vi "Analog Read Benchmark.vi"(0 "Stop Button":bool, 11 "AO Channels":u8[](array[numeric])=[0, 0, 0, 0, 0, 0, 0, 0, 0, 0, 0, 0]) -> (2 "Voltages":dbl[](array[numeric]), 3 "Loop Time (ms)":i32, 6 "Loop Rate":dbl(graph), 7 "Device Name":string)   [LabVIEW 2013]
uses:
  <vilib>/LabVIEW Hacker/LINX/Private/Type Defs/Interface.ctl
  <vilib>/LabVIEW Hacker/LINX/Private/Device/Type Defs/TCP Config.ctl
  <vilib>/LabVIEW Hacker/LINX/Private/Device/Device.lvlib
  <vilib>/LabVIEW Hacker/LINX/LVH-LINX.lvlib
  <vilib>/ptbypt/NI_PtbyPt.lvlib
panel:
  out "Voltages":dbl[](graph)
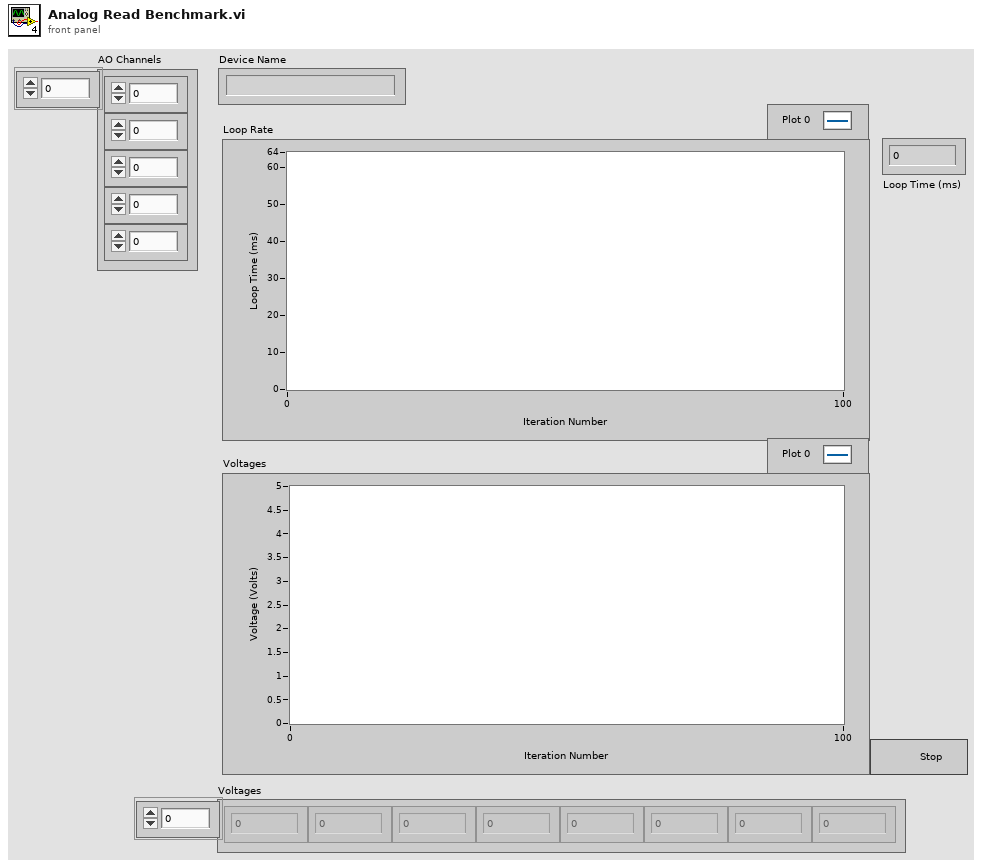
[diagram p1: front panel]
types:
  T1 = typedef "LVH-LINX.lvlib/Device.lvlib/TCP Config.ctl" = cluster{"IP Address":string, "Port":u16}
  T2 = typedef "LVH-LINX.lvlib/Interface.ctl" = enum16{"Serial", "TCP"}
  T3 = typedef "LVH-LINX.lvlib/Device.lvlib/LINX Device Config.ctl" = cluster{"Interface":T2, "COM Port":refnum<visa-resource-name>, "TCP Configuration":T1, "Device Family":T4, "Device ID":u8, "Device Name":string, "TCP Ref":refnum<k5>}
  T4 = typedef "LVH-LINX.lvlib/Device Family.ctl" = enum8{"National Instruments", "Digilent", "Arduino"}
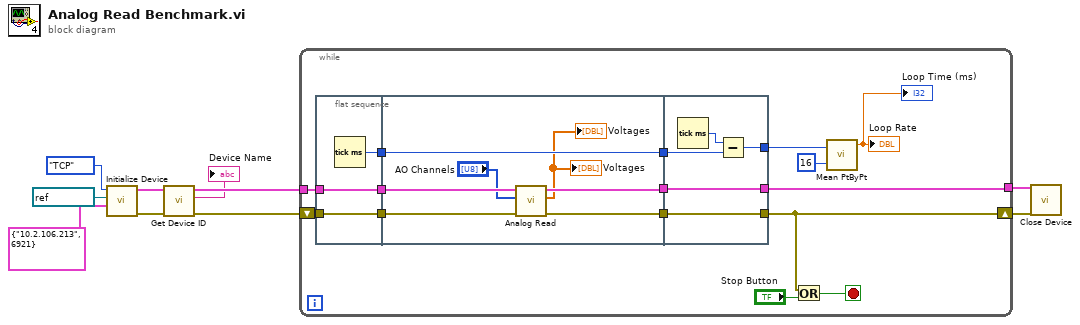
[diagram p0: block diagram]
diagram:
  n1 = call <vilib>:"Initialize Device.vi"("TCP Configuration"=T1 {"IP Address"="10.2.106.213", "Port"=6921}, "COM Port"=refnum<visa-resource-name> "COM5", "Interface"=Interface."TCP") -> ("Error Out"=w6:errorcluster, "LINX Device Config"=w7:T3)  [unwired: 6 in, 1 out]
  n2 = call <vilib>:"Get Device ID.vi"("Error In"=w6, "LINX Device Config"=w7) -> ("Error Out"=w5:errorcluster, "Device Name"=→"Device Name":string, "LINX Device Config"=w4:T3)  [unwired: 7 in]
  n3 = while {
    tunnel: w4 -> [w25]
    shift-right: [w11] -> w8
    shift-left: w5 -> [w13]
    tunnel: [w16] -> w2
    stop <- w24 stop-if-true
    n4 = flat-sequence {
      tunnel: w25 -> [w28]
      tunnel: [w28] -> w22
      tunnel: [w27] -> w21
      tunnel: w13 -> [w26]
      tunnel: [w26] -> w12
      tunnel: w22 -> [w34]
      tunnel: w21 -> [w35]
      tunnel: [w35] -> w20
      tunnel: [w33] -> w15
      tunnel: [w32] -> w14
      tunnel: w12 -> [w31]
      tunnel: w20 -> [w39]
      tunnel: [w38] -> w19
      tunnel: [w37] -> w16
      tunnel: w15 -> [w37]
      tunnel: w14 -> [w36]
      tunnel: [w36] -> w11
      frame #0 {
        n5 = Tick Count (ms)() -> (millisecond timer value=w27:u32)
      }
      frame #1 {
        n6 = call <vilib>:"Analog Read.vi"("Error In"=w31, "AI Channels"="AO Channels", "LINX Device Config"=w34) -> ("Error Out"=w32:errorcluster, "Voltages"=→"Voltages" →"Voltages":dbl[], "LINX Device Config"=w33:T3)  [unwired: 5 in, 1 out]
      }
      frame #2 {
        n7 = Tick Count (ms)() -> (millisecond timer value=w40:u32)
        n8 = Subtract(x=w40, y=w39) -> (x-y=w38:u32)
      }
    }
    n9 = Or(x=w11, y="Stop Button") -> (x .or. y?=w24:bool)
    n10 = call <vilib>:"Mean PtByPt.vi"("x"=w19, "sample length"=16) -> ("mean"=→"Loop Rate" →"Loop Time (ms)":dbl)  [unwired: 2 in, 1 out]
  }
  n11 = call <vilib>:"Close Device.vi"("Error In"=w8, "LINX Device Config"=w2) -> ()  [unwired: 8 in, 2 out]
